vi "labview_pid.vi"() -> ()   [LabVIEW 2019]
panel:
  out "return value":dbl[](array[numeric])
  in  "stop":bool
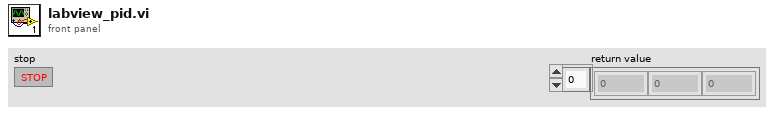
[diagram p1: front panel]
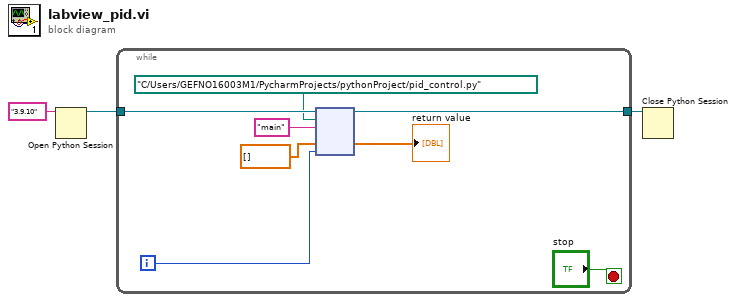
[diagram p0: block diagram]
diagram:
  n1 = Open Python Session(python version="3.9.10" ("Python version")) -> (session out=w3:refnum<k35>)  [unwired: 2 in, 1 out]
  n2 = while {
    tunnel: w3 -> [w11]
    tunnel: [w10] -> w2
    i -> [w6]
    stop <- "stop" stop-if-true
    n3 = node(w11, path "C:/Users/GEFNO16003M1/PycharmProjects/pythonProject/pid_control.py" ("module path"), "main" ("function name"), dbl[] [], w6) -> (w10:refnum<k35>, →"return value":dbl[])  [unwired: 2 in, 3 out]
  }
  n4 = Close Python Session(session in=w2) -> ()  [unwired: 1 in, 1 out]
